vi "Burst XCtl Test.vi"() -> ()   [LabVIEW 2015]
uses:
  XControls/Burst (G3)/Burst Data.ctl
  XControls/Burst (G3)/Burst (G3).xctl
panel:
  out "Array Out":T1[](array[typedef])
  in  "Burst (G3)":T2(xcontrol)
  in  "Array":T1[](array[typedef])=[{"Active"=TRUE, "Delay (ms)"=0.0, "Duration (ms)"=50.0, "Ramp (ms)"=5.0, "Rate (Hz)"=0.0, "Trepeat (ms)"=0.0, "Repeat"=FALSE}, {"Active"=TRUE, "Delay (ms)"=0.0, "Duration (ms)"=50.0, "Ramp (ms)"=5.0, "Rate (Hz)"=0.0, "Trepeat (ms)"=0.0, "Repeat"=FALSE}]
  in  "Apply":bool
  in  "stop":bool
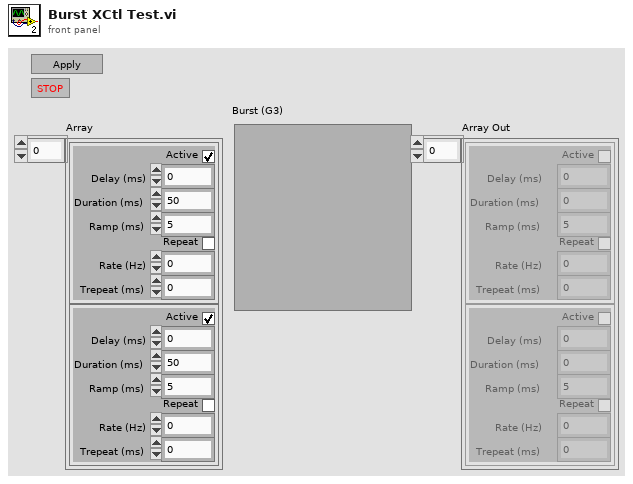
[diagram p1: front panel]
types:
  T1 = typedef "Burst (G3).xctl/Burst Data.ctl" = cluster{"Active":bool, "Delay (ms)":dbl, "Duration (ms)":dbl, "Ramp (ms)":dbl, "Rate (Hz)":dbl, "Trepeat (ms)":dbl, "Repeat":bool}
  T2 = cluster{"Active":bool, "Delay (ms)":dbl, "Duration (ms)":dbl, "Ramp (ms)":dbl, "Rate (Hz)":dbl, "Trepeat (ms)":dbl, "Repeat":bool}
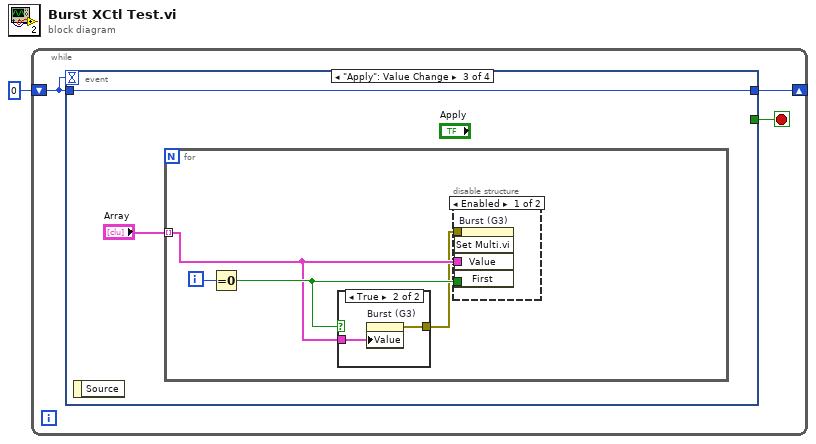
[diagram p0: block diagram]
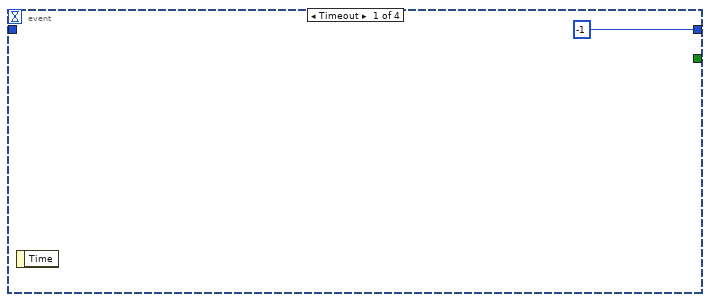
[diagram p2: hidden frame]
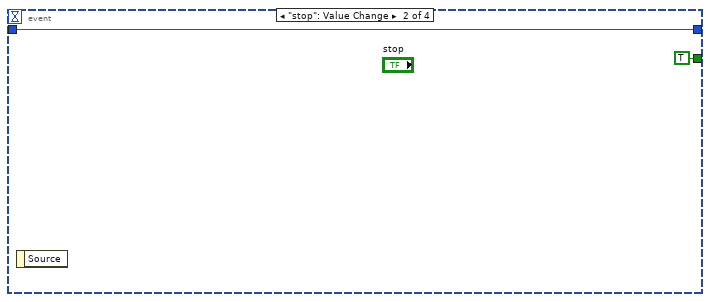
[diagram p3: hidden frame]
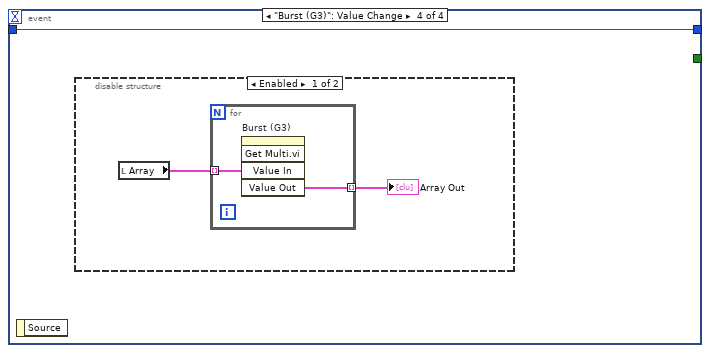
[diagram p6: hidden frame]
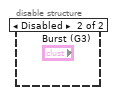
[diagram p7: hidden frame]
diagram:
  n1 = while {
    shift-right: [w2] -> _
    shift-left: 0 -> [w3]
    stop <- w4 stop-if-true
    n2 = event shown="[2] \"Apply\": Value Change" {
      selector: _ -> [_ _ _ _]
      dyn-events: _ -> [_ _ _ _]
      timeout: w3 -> [_ _ _ _]
      tunnel: [_ TRUE _ _] -> w4
      tunnel: w3 -> [_ w6 w9 w19]
      tunnel: [-1 w6 w9 w19] -> w2
      event Timeout {
        n3 = event-data() -> ()  [unwired: 1 in, 1 out]
      }
      event "stop": Value Change {
        n4 = event-data() -> ()  [unwired: 1 in, 1 out]
      }
      event "Apply": Value Change {
        n5 = event-data() -> ()  [unwired: 1 in, 1 out]
        n6 = for {
          tunnel: "Array" -> [w11] mode=indexing
          i -> [w13]
          n7 = Equal To 0?(x=w13) -> (x = 0?=w12:bool)
          n8 = case shown="True" w12 {
            tunnel: w11 -> [_ w18]
            tunnel: [_ w17] -> w10
            frame False {
            }
            frame True {
              n9 = property on="Burst (G3)" class="Burst (G3) (strict)"("Value"=w18) -> (error out=w17:errorcluster)  [unwired: 2 in, 1 out]
            }
          }
          n10 = disable-structure shown="Enabled" {
            disable-tunnel: w12 -> [w16 _]
            disable-tunnel: w11 -> [w15 _]
            disable-tunnel: w10 -> [w14 _]
            frame Enabled {
              n11 = invoke on="Burst (G3)" class="Burst (G3) (strict)" method="Set Multi.vi"(error in=w14, "Value"=w15, "First"=w16) -> ()  [unwired: 2 in, 5 out]
            }
            frame Disabled {
            }
          }
        }
      }
      event "Burst (G3)": Value Change {
        n12 = event-data() -> ()  [unwired: 1 in, 1 out]
        n13 = disable-structure shown="Enabled" {
          frame Enabled {
            n14 = local read "Array"() -> (w21:T1[])
            n15 = for {
              tunnel: w21 -> [w23] mode=indexing
              tunnel: [w22] -> w20 mode=indexing
              n16 = invoke on="Burst (G3)" class="Burst (G3) (strict)" method="Get Multi.vi"("Value In"=w23) -> ("Value Out"=w22:T1)  [unwired: 4 in, 4 out]
            }
            "Array Out" <- w20
          }
          frame Disabled {
          }
        }
      }
    }
  }
